vi "SaveTdms.vi"(0 "object in":refnum<class "MTec.lvclass">, 2 "tdms file":refnum<k34>, 3 "group name":string, 5 "error in (no error)":errorcluster) -> (14 "object out":refnum<class "MTec.lvclass">, 16 "MtecData":T3={"meTEC_CH2_Temperature Stability"=1, "meTEC_CH2_Act. Output Current [A]"=0.0, "meTEC_CH2_Act. Output Voltage [V]"=0.0, "meTEC_CH2_Object Temperature [°C]"=0.0, "meTEC_CH2_Sink Temperature [°C]"=0.0, "meTEC_CH1_Error Parameter"=0, "meTEC_CH1_Error Instance"=0, "meTEC_CH1_Error No."=0, "meTEC_CH1_Device Status"=1, "meTEC_CH1_Temperature Stability"=1, "meTEC_CH1_Act. Output Current [A]"=0.0, "meTEC_CH1_Act. Output Voltage [V]"=0.0, "meTEC_CH1_Object Temperature [°C]"=0.0, "meTEC_CH1_Sink Temperature [°C]"=0.0} {"meTEC_CH1_Sink Temperature [°C]" format="%.3f"; "meTEC_CH1_Object Temperature [°C]" format="%.3f"; "meTEC_CH1_Act. Output Voltage [V]" format="%.3f"; "meTEC_CH1_Act. Output Current [A]" format="%.3f"; "meTEC_CH1_Temperature Stability" items=["Temperature regulation is not active", "Is not stable", "Is stable"]; "meTEC_CH1_Device Status" items=["Initializing", "Ready", "Run", "Error", "Bootloader", "Reset in Progress"]; "meTEC_CH2_Sink Temperature [°C]" format="%.3f"; "meTEC_CH2_Object Temperature [°C]" format="%.3f"; "meTEC_CH2_Act. Output Voltage [V]" format="%.3f"; "meTEC_CH2_Act. Output Current [A]" format="%.3f"; "meTEC_CH2_Temperature Stability" items=["Temperature regulation is not active", "Is not stable", "Is stable"]}, 19 "error out":errorcluster)   [LabVIEW 2019, in "MTec.lvclass"]
uses:
  MTec.lvclass
  TEC LabVIEW Control Software v0.14/Source/LV Source/[meerstetter engineering TE Cooling]/TypeDefs/meTEC_ID 1200_Temperature is Stable.ctl
  TEC LabVIEW Control Software v0.14/Source/LV Source/[meerstetter engineering TE Cooling]/TypeDefs/meTEC_ID 104_Device Status.ctl
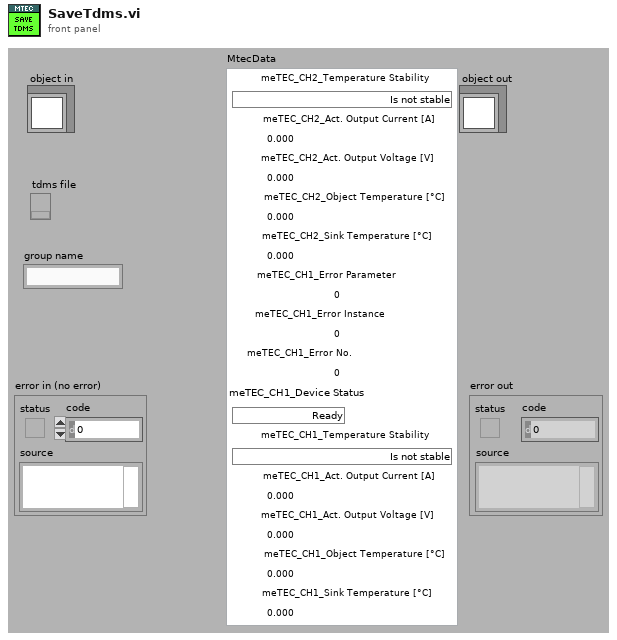
[diagram p1: front panel]
types:
  T1 = typedef "meTEC_ID 1200_Temperature is Stable.ctl" = i32
  T2 = typedef "meTEC_ID 104_Device Status.ctl" = i32
  T3 = cluster{"meTEC_CH2_Temperature Stability":T1, "meTEC_CH2_Act. Output Current [A]":dbl, "meTEC_CH2_Act. Output Voltage [V]":dbl, "meTEC_CH2_Object Temperature [°C]":dbl, "meTEC_CH2_Sink Temperature [°C]":dbl, "meTEC_CH1_Error Parameter":i32, "meTEC_CH1_Error Instance":i32, "meTEC_CH1_Error No.":i32, "meTEC_CH1_Device Status":T2, "meTEC_CH1_Temperature Stability":T1, "meTEC_CH1_Act. Output Current [A]":dbl, "meTEC_CH1_Act. Output Voltage [V]":dbl, "meTEC_CH1_Object Temperature [°C]":dbl, "meTEC_CH1_Sink Temperature [°C]":dbl}
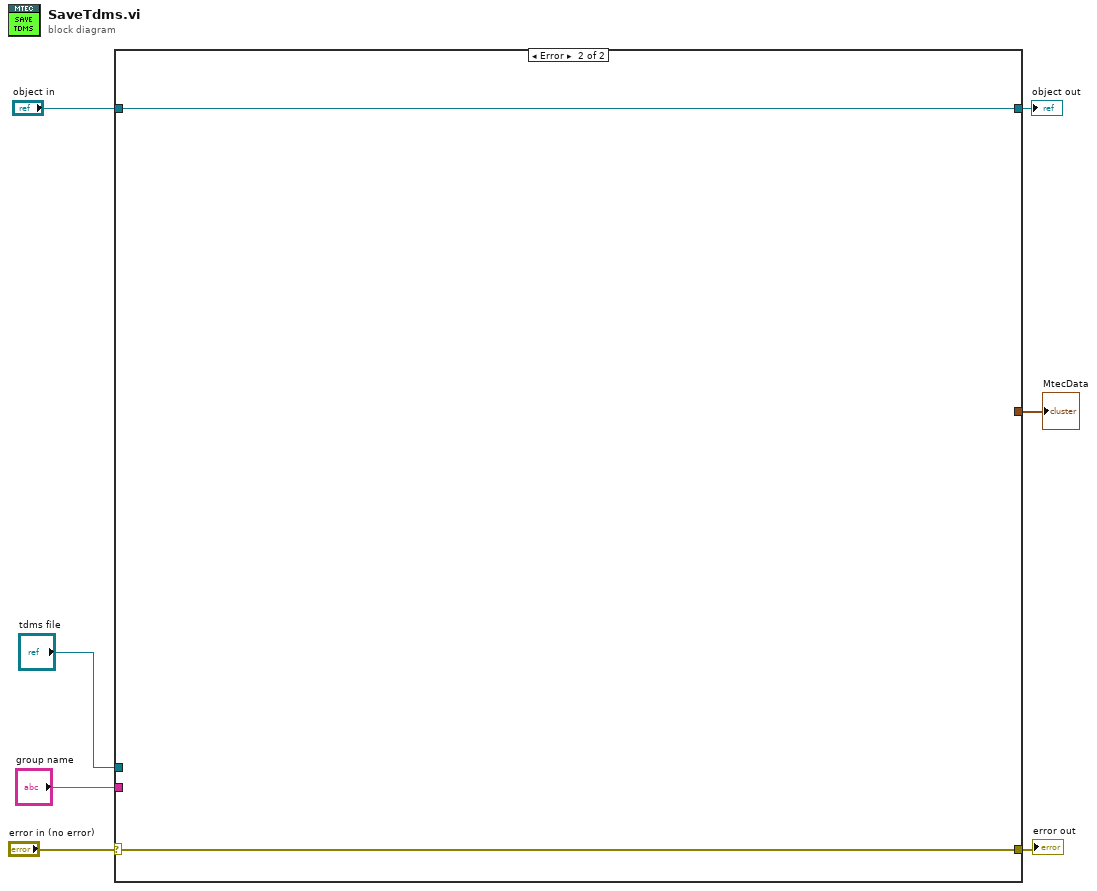
[diagram p0: block diagram]
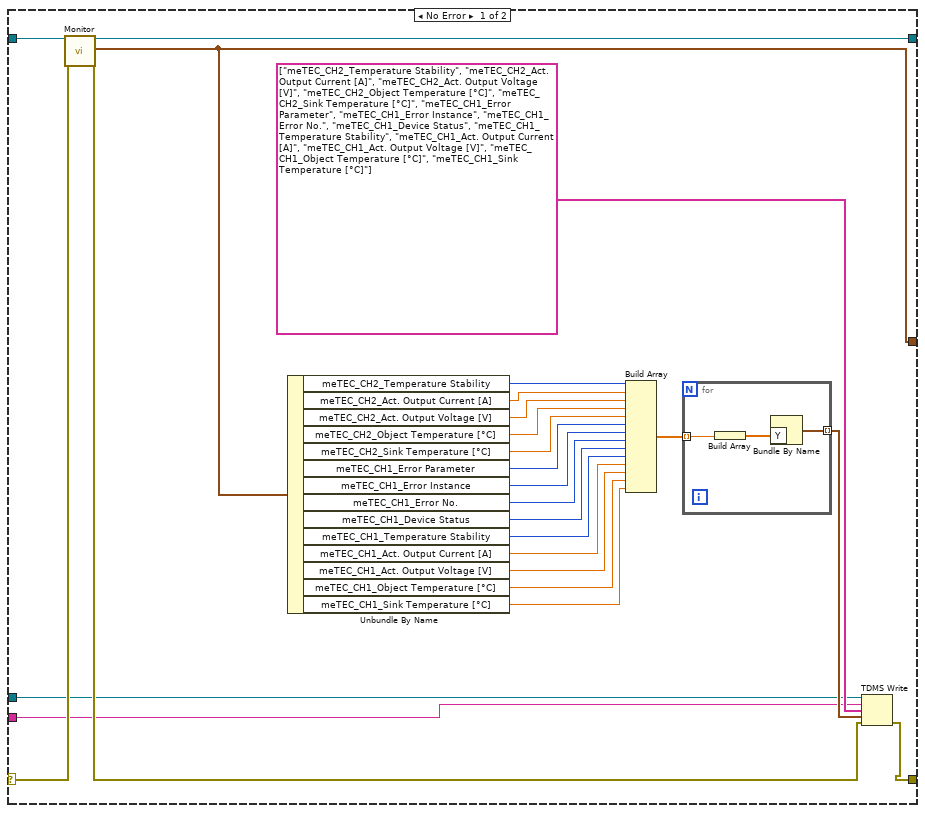
[diagram p2: hidden frame]
diagram:
  n1 = case shown="Error" "error in (no error)" {
    selector: "error in (no error)" -> [w16 w37]
    tunnel: [w11 w37] -> w6
    tunnel: [w18 w36] -> w4
    tunnel: "object in" -> [w17 w36]
    tunnel: "tdms file" -> [w10 _]
    tunnel: "group name" -> [w9 _]
    tunnel: [w8 _] -> w1
    frame No Error {
      n2 = call-dynamic "Monitor.vi"("object in"=w17, "error in (no error)"=w16) -> ("object out"=w18:refnum<class "MTec.lvclass">, "MtecData"=w8:T3, "error out"=w12:errorcluster)  [unwired: 15 in]
      n3 = Unbundle By Name(w8) -> ("meTEC_CH2_Temperature Stability"=w32:T1, "meTEC_CH2_Act. Output Current [A]"=w31:dbl, "meTEC_CH2_Act. Output Voltage [V]"=w30:dbl, "meTEC_CH2_Object Temperature [°C]"=w29:dbl, "meTEC_CH2_Sink Temperature [°C]"=w28:dbl, "meTEC_CH1_Error Parameter"=w27:i32, "meTEC_CH1_Error Instance"=w26:i32, "meTEC_CH1_Error No."=w25:i32, "meTEC_CH1_Device Status"=w24:T2, "meTEC_CH1_Temperature Stability"=w23:T1, "meTEC_CH1_Act. Output Current [A]"=w22:dbl, "meTEC_CH1_Act. Output Voltage [V]"=w21:dbl, "meTEC_CH1_Object Temperature [°C]"=w20:dbl, "meTEC_CH1_Sink Temperature [°C]"=w19:dbl)
      n4 = Build Array(w32, w31, w30, w29, w28, w27, w26, w25, w24, w23, w22, w21, w20, w19) -> (w15:dbl[])
      n5 = for {
        tunnel: w15 -> [w35] mode=indexing
        tunnel: [w33] -> w14 mode=indexing
        n6 = Build Array(w35) -> (w34:dbl[])
        n7 = Bundle By Name("Y"=w34) -> (w33:waveform(dbl))  [unwired: 1 in]
      }
      n8 = TDMS Write(0:w10, 5:w9, 7:string[] ["meTEC_CH2_Temperature Stability", "meTEC_CH2_Act. Output Current [A]", "meTEC_CH2_Act. Output Voltage [V]", "meTEC_CH2_Object Temperature [°C]", "meTEC_CH2_Sink Temperature [°C]", "meTEC_CH1_Error Parameter", "meTEC_CH1_Error Instance", "meTEC_CH1_Error No.", "meTEC_CH1_Device Status", "meTEC_CH1_Temperature Stability", "meTEC_CH1_Act. Output Current [A]", "meTEC_CH1_Act. Output Voltage [V]", "meTEC_CH1_Object Temperature [°C]", "meTEC_CH1_Sink Temperature [°C]"] ("Array"), 9:w14, 11:w12) -> (15:w11:errorcluster)  [unwired: 1 in, 3 out]
    }
    frame Error {
    }
  }
  "error out" <- w6
  "object out" <- w4
  "MtecData" <- w1
